vi "SV Histogram.vi"   [LabVIEW 2017]
doc: "Use this VI to create a histogram of the input data. Set <B>range</B> and <B>number of bins</B> to specify the bins to include. Choose the appropriate instance based on the input data."
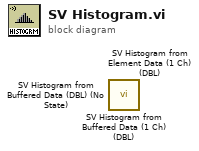
[diagram p0: block diagram]
diagram:
  n1 = call <vilib>:"SV Histogram from Buffered Data (1 Ch) (DBL).vi"() -> ()  [unwired: 13 in, 3 out]
  n2 = call <vilib>:"SV Histogram from Element Data (1 Ch) (DBL).vi"() -> ()  [unwired: 13 in, 3 out]
  n3 = call <vilib>:"SV Histogram from Buffered Data (DBL) (No State).vi"() -> ()  [unwired: 13 in, 3 out]
